vi "Hex to Normal String.vi"(1 "Hex In":string) -> (0 "Normal Array Out":string[](array[string]))   [LabVIEW 2014, in "StringConvert.lvlib"]
uses:
  StringConvert.lvlib
panel:
  out "Normal Out":string
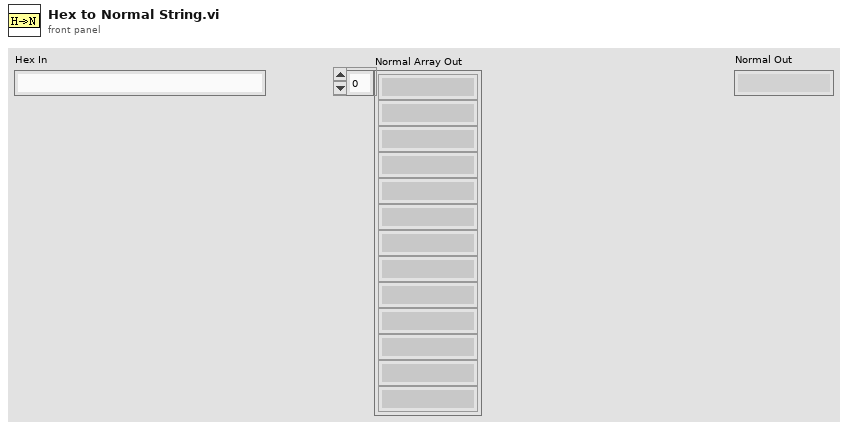
[diagram p1: front panel]
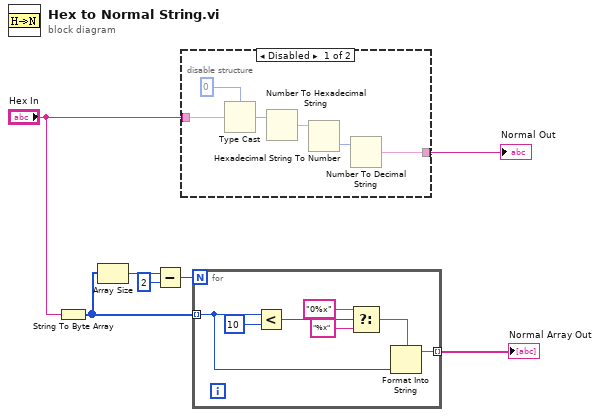
[diagram p0: block diagram]
diagram:
  n1 = String To Byte Array(string="Hex In") -> (unsigned byte array=w4:u8[])
  n2 = Array Size(array=w4) -> (size(s)=w2:i32)
  n3 = Subtract(x=w2, y=2) -> (x-y=w3:i32)
  n4 = disable-structure shown="Disabled" {
    disable-tunnel: [w9 w14] -> w7
    disable-tunnel: "Hex In" -> [w8 w14]
    frame Disabled {
      n5 = Type Cast(type=u16 0, x=w8) -> (*(type *) &x=w12:u16)
      n6 = Number To Hexadecimal String(2:w12) -> (0:w11:string)  [unwired: 1 in]
      n7 = Hexadecimal String To Number(string=w11) -> (number=w10:u32)  [unwired: 2 in, 1 out]
      n8 = Number To Decimal String(number=w10) -> (decimal integer string=w9:string)  [unwired: 1 in]
    }
    frame Enabled {
    }
  }
  "Normal Out" <- w7
  n9 = for {
    N: w3 -> [_]
    tunnel: w4 -> [w16] mode=indexing
    tunnel: [w15] -> w5 mode=indexing
    n10 = Less?(x=w16, y=u8 10) -> (x < y?=w20:bool)
    n11 = Select(t="0%x", s=w20, f="%x") -> (s? t:f=w19:string)
    n12 = Format Into String(format string=w19, w16) -> (resulting string=w15:string)  [unwired: 2 in, 1 out]
  }
  "Normal Array Out" <- w5
